vi "TDC_clearAllHistograms.vi"(8 "Error In":errorcluster) -> (0 "Error Out":errorcluster)   [LabVIEW 2011]
uses:
  tdcbase.dll
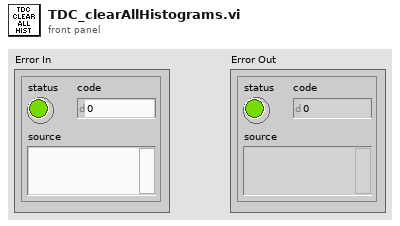
[diagram p1: front panel]
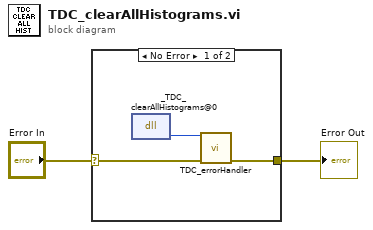
[diagram p0: block diagram]
diagram:
  n1 = case shown="No Error" "Error In" {
    selector: "Error In" -> [w3 w6]
    tunnel: [w4 w6] -> w2
    frame No Error {
      n2 = dll-call lib="X:/tdcbase.dll" fn="_TDC_clearAllHistograms@0"() -> ("return type"=w5:i32)  [unwired: 3 in, 2 out]
      n3 = call "TDC_errorHandler.vi"("Error In"=w3, "TDC Return Code"=w5) -> ("Error Out"=w4:errorcluster)  [unwired: 9 in]
    }
    frame Error {
    }
  }
  "Error Out" <- w2
